vi "Launch-plant.vi"(8 "error in (no error)":errorcluster, 10 "Plant VI path":path=path "C:/ni-rt/startup/Plant1.vi", 11 "Machine IP Address":string="193.0.0.2") -> (0 "error out":errorcluster={"status"=TRUE, "code"=7, "source"="Open VI Reference in Launch-plant.vi<APPEND>\n<b>C:\\ni-rt\\Run-plant.vi</b>"}, 3 "Plant VI reference out":refnum<vi>)   [LabVIEW 2016]
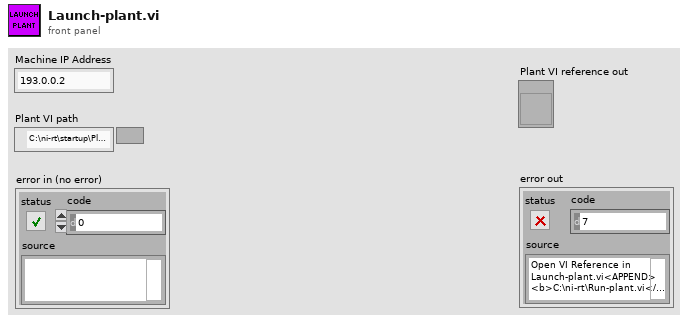
[diagram p1: front panel]
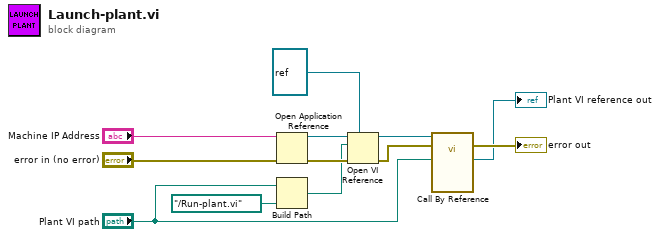
[diagram p0: block diagram]
diagram:
  n1 = Open Application Reference(8:"error in (no error)", 11:"Machine IP Address") -> (0:w12:errorcluster, 3:w10:refnum<vi>)  [unwired: 2 in]
  n2 = Build Path(base path="Plant VI path", name or relative path=path "../Run-plant.vi") -> (appended path=w2:path)
  n3 = Open VI Reference(type specifier VI Refnum (for type only)=refnum<vi> refnum, application reference (local)=w10, vi path=w2, error in (no error)=w12) -> (vi reference=w6:refnum<vi>, error out=w9:errorcluster)  [unwired: 2 in]
  n4 = call-by-ref "?"(reference=w6, error in=w9, "Plant VI path"="Plant VI path") -> (error out=→"error out":errorcluster, "reference out"=→"Plant VI reference out":refnum<vi>)  [unwired: 9 in, 2 out]
